vi "XL320_Send Direct Command.vi"(0 "VISA resource name":refnum<visa-resource-name>, 1 "Select Action":T1=3 items=["Ping"=1, "Read"=2, "Write"=3, "Registered Write"=4, "Action"=5, "Reset"=6, "Reboot"=8, "Status"=85, "Sync Read"=130, "Sync Write"=131, "Bulk Read"=146, "Bulk Write"=147], 2 "Motor ID (0)":u8, 3 "Address":u16, 4 "Parameters":string, 5 "Error in (no error)":errorcluster) -> (14 "VISA resource name out":refnum<visa-resource-name>, 17 "Command to Serial":string, 19 "Error out":errorcluster)   [LabVIEW 2017, in "Dynamixel XL320.lvlib"]
doc: "Using any of the six basic commands for the Dynamixel motor, this VI allows you to send any set of parameters to the motor(s). This is a Low-Level VI that is used by other VIs."
uses:
  <instrlib>/Dynamixel XL320 (Drivers instrument)/Dynamixel XL320.lvlib
  <instrlib>/Dynamixel XL320 (Drivers instrument)/Public/Configure/XL320_Select_Action.ctl
panel:
  # "Ghislain REMY, IUT de Cachan, 2015 December 2015"
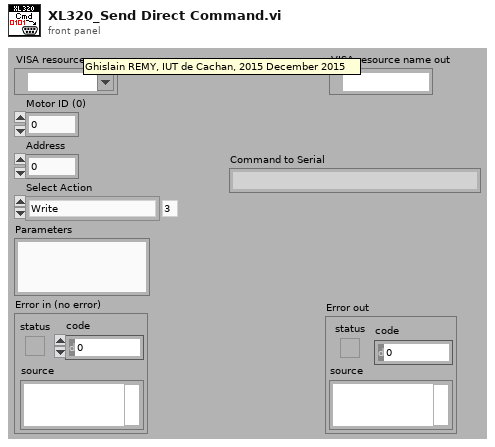
[diagram p1: front panel]
types:
  T1 = typedef "Dynamixel XL320.lvlib/XL320_Select_Action.ctl" = u8
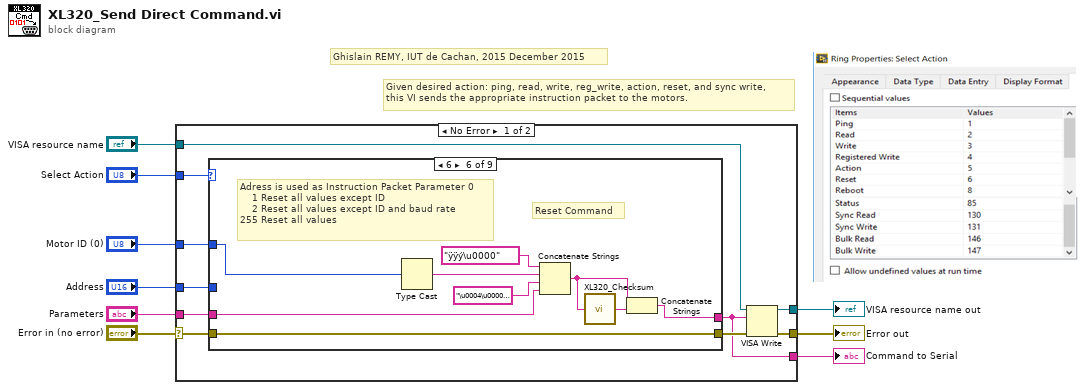
[diagram p0: block diagram]
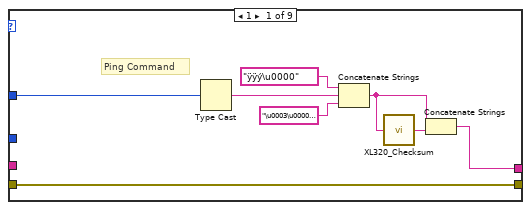
[diagram p2: hidden frame]
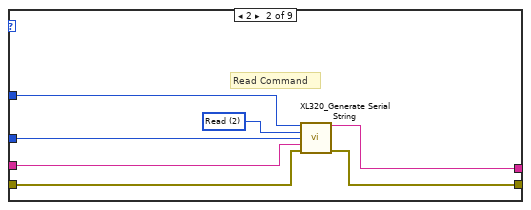
[diagram p3: hidden frame]
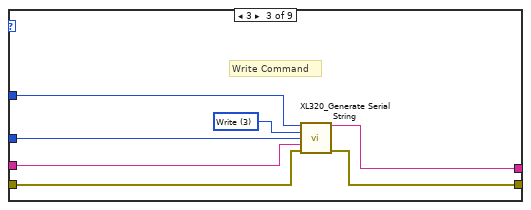
[diagram p4: hidden frame]
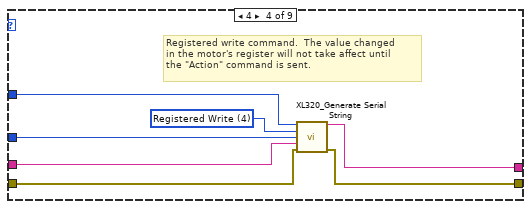
[diagram p5: hidden frame]
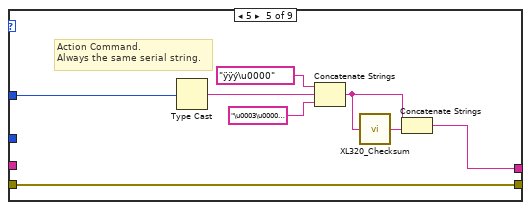
[diagram p6: hidden frame]
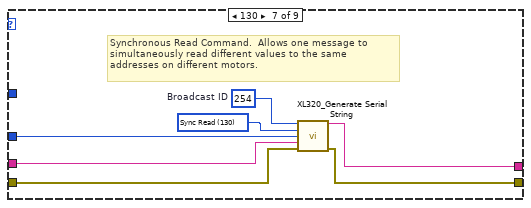
[diagram p7: hidden frame]
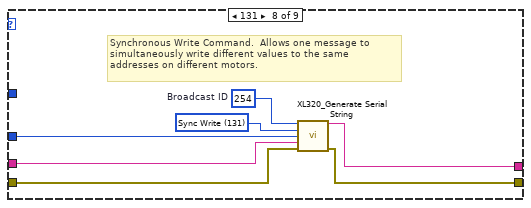
[diagram p8: hidden frame]
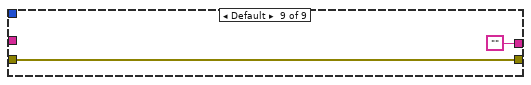
[diagram p9: hidden frame]
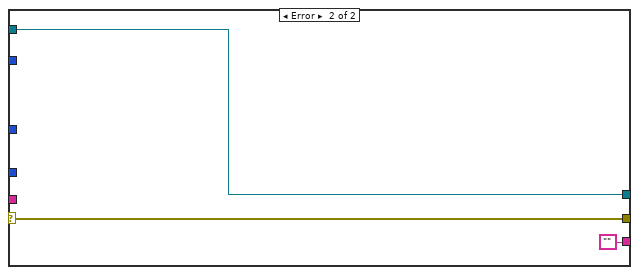
[diagram p10: hidden frame]
diagram:
  # "Ghislain REMY, IUT de Cachan, 2015 December 2015"
  # "Given desired action: ping, read, write, reg_write, action, reset, and sync write,\nthis VI sends the appropriate instruction packet to the motors."
  n1 = case shown="No Error" "Error in (no error)" {
    selector: "Error in (no error)" -> [w15 w84]
    tunnel: "Parameters" -> [w19 _]
    tunnel: "Address" -> [w18 _]
    tunnel: "Motor ID (0)" -> [w17 _]
    tunnel: "Select Action" -> [w16 _]
    tunnel: [w12 w84] -> w7
    tunnel: [w14 w83] -> w6
    tunnel: "VISA resource name" -> [w11 w83]
    tunnel: [w10 ""] -> w2
    frame No Error {
      n2 = case shown="6" w16 {
        tunnel: w15 -> [w23 w31 w38 w45 w56 w59 w69 w76 w80]
        tunnel: [w23 w30 w37 w43 w56 w59 w68 w75 w80] -> w13
        tunnel: w17 -> [w25 w34 w41 w48 w50 w58 _ _ _]
        tunnel: w18 -> [_ w33 w40 w47 _ _ w71 w78 _]
        tunnel: w19 -> [_ w32 w39 w46 _ w57 w70 w77 _]
        tunnel: [w21 w29 w36 w44 w49 w60 w67 w74 ""] -> w10
        frame 1 {
          # "Ping Command"
          n3 = Type Cast(x=w25) -> (*(type *) &x=w24:string)  [unwired: 1 in]
          n4 = Concatenate Strings("ÿÿý\u0000", w24, "\u0003\u0000\u0001") -> (w20:string)
          n5 = call <instrlib>:"XL320_Checksum.vi"("Input String"=w20) -> ("Checksum String"=w22:string)
          n6 = Concatenate Strings(w20, w22) -> (w21:string)
        }
        frame 2 {
          w28 = T1 2 items=["Ping"=1, "Read"=2, "Write"=3, "Registered Write"=4, "Action"=5, "Reset"=6, "Reboot"=8, "Status"=85, "Sync Read"=130, "Sync Write"=131, "Bulk Read"=146, "Bulk Write"=147] ("Select Action")
          # "Read Command"
          n7 = call <instrlib>:"XL320_Generate Serial String.vi"("Motor ID"=w34, "Select Action"=w28, "Address"=w33, "Parameters"=w32, "Error in (no error)"=w31) -> ("Command to Serial"=w29:string, "error out"=w30:errorcluster)  [unwired: 9 in]
        }
        frame 3 {
          w35 = T1 3 items=["Ping"=1, "Read"=2, "Write"=3, "Registered Write"=4, "Action"=5, "Reset"=6, "Reboot"=8, "Status"=85, "Sync Read"=130, "Sync Write"=131, "Bulk Read"=146, "Bulk Write"=147] ("Select Action")
          # "Write Command"
          n8 = call <instrlib>:"XL320_Generate Serial String.vi"("Motor ID"=w41, "Select Action"=w35, "Address"=w40, "Parameters"=w39, "Error in (no error)"=w38) -> ("Command to Serial"=w36:string, "error out"=w37:errorcluster)  [unwired: 9 in]
        }
        frame 4 {
          w42 = T1 4 items=["Ping"=1, "Read"=2, "Write"=3, "Registered Write"=4, "Action"=5, "Reset"=6, "Reboot"=8, "Status"=85, "Sync Read"=130, "Sync Write"=131, "Bulk Read"=146, "Bulk Write"=147] ("Select Action")
          # "Registered write command.  The value changed \nin the motor's register will not take affect until \nthe \"Action\" command is sent."
          n9 = call <instrlib>:"XL320_Generate Serial String.vi"("Motor ID"=w48, "Select Action"=w42, "Address"=w47, "Parameters"=w46, "Error in (no error)"=w45) -> ("Command to Serial"=w44:string, "error out"=w43:errorcluster)  [unwired: 9 in]
        }
        frame 5 {
          # "Action Command.\nAlways the same serial string."
          n10 = Type Cast(x=w50) -> (*(type *) &x=w54:string)  [unwired: 1 in]
          n11 = Concatenate Strings("ÿÿý\u0000", w54, "\u0003\u0000\u0005") -> (w52:string)
          n12 = call <instrlib>:"XL320_Checksum.vi"("Input String"=w52) -> ("Checksum String"=w53:string)
          n13 = Concatenate Strings(w52, w53) -> (w49:string)
        }
        frame 6 {
          # "Adress is used as Instruction Packet Parameter 0\n    1 Reset all values except ID\n    2 Reset all values except ID and baud rate\n255 Reset all values"
          # "Reset Command"
          n14 = Type Cast(x=w58) -> (*(type *) &x=w64:string)  [unwired: 1 in]
          n15 = Concatenate Strings("ÿÿý\u0000", w64, "\u0004\u0000\u0006", w57) -> (w62:string)
          n16 = call <instrlib>:"XL320_Checksum.vi"("Input String"=w62) -> ("Checksum String"=w63:string)
          n17 = Concatenate Strings(w62, w63) -> (w60:string)
        }
        frame 130 {
          w66 = T1 130 items=["Ping"=1, "Read"=2, "Write"=3, "Registered Write"=4, "Action"=5, "Reset"=6, "Reboot"=8, "Status"=85, "Sync Read"=130, "Sync Write"=131, "Bulk Read"=146, "Bulk Write"=147] ("Select Action")
          w72 = u8 254  # Broadcast ID
          # "Synchronous Read Command.  Allows one message to\nsimultaneously read different values to the same \naddresses on different motors."
          n18 = call <instrlib>:"XL320_Generate Serial String.vi"("Motor ID"=w72, "Select Action"=w66, "Address"=w71, "Parameters"=w70, "Error in (no error)"=w69) -> ("Command to Serial"=w67:string, "error out"=w68:errorcluster)  [unwired: 9 in]
        }
        frame 131 {
          w73 = T1 131 items=["Ping"=1, "Read"=2, "Write"=3, "Registered Write"=4, "Action"=5, "Reset"=6, "Reboot"=8, "Status"=85, "Sync Read"=130, "Sync Write"=131, "Bulk Read"=146, "Bulk Write"=147] ("Select Action")
          w79 = u8 254  # Broadcast ID
          # "Synchronous Write Command.  Allows one message to\nsimultaneously write different values to the same \naddresses on different motors."
          n19 = call <instrlib>:"XL320_Generate Serial String.vi"("Motor ID"=w79, "Select Action"=w73, "Address"=w78, "Parameters"=w77, "Error in (no error)"=w76) -> ("Command to Serial"=w74:string, "error out"=w75:errorcluster)  [unwired: 9 in]
        }
        frame Default {
        }
      }
      n20 = VISA Write(VISA resource name=w11, write buffer=w10, error in (no error)=w13) -> (VISA resource name out=w14:refnum<visa-resource-name>, error out=w12:errorcluster)  [unwired: 1 out]
    }
    frame Error {
    }
  }
  "Error out" <- w7
  "VISA resource name out" <- w6
  "Command to Serial" <- w2
